vi "按修改时间读取文件夹下文件.vi"(8 "error in (no error)":errorcluster caption="错误输入（无错误）", 11 "路径":path) -> (0 "error out":errorcluster caption="错误输出", 3 "文件名":string[](array[string]))   [LabVIEW 2013]
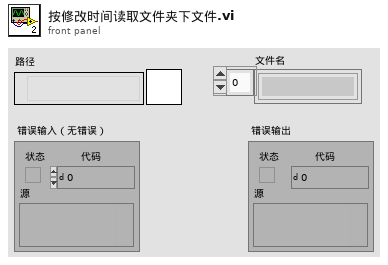
[diagram p1: front panel]
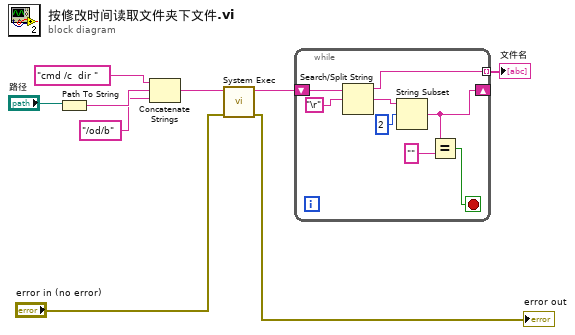
[diagram p0: block diagram]
diagram:
  n1 = Path To String(path="路径") -> (string=w7:string)
  n2 = Concatenate Strings("cmd /c  dir ", w7, "/od/b" ("字符串")) -> (w5:string)
  n3 = call <vilib>:"System Exec.vi"("error in (no error)"="error in (no error)", "command line"=w5) -> ("error out"=→"error out":errorcluster, "standard output"=w4:string)  [unwired: 6 in, 2 out]
  n4 = while {
    shift-right: [w13] -> _
    shift-left: w4 -> [w17]
    tunnel: [w15] -> w3 mode=indexing
    stop <- w11 stop-if-true
    n5 = Search/Split String(string=w17, search string/char (-)="\r") -> (substring before match=w15:string, match + rest of string=w14:string)  [unwired: 1 in, 1 out]
    n6 = String Subset(string=w14, offset (0)=2 ("长度（剩余）")) -> (substring=w13:string)  [unwired: 1 in]
    n7 = Equal?(x=w13, y="") -> (x = y?=w11:bool)
  }
  "文件名" <- w3
